vi "SelectColumnstoPlaybackDisplay_171213.vi"(11 "Clean data array in":dbl[][](array[numeric])) -> (0 "Speed":dbl[](array[numeric]), 1 "TotalDIstanceTraveled":dbl, 2 "Playbackprogress(min)maxscale":dbl, 3 "CurrentDIstancemaxScale":dbl, 4 "AVGSpeed":dbl, 5 "CurrentDistanceTraveled":dbl[](array[numeric]), 6 "TTL":dbl[](array[numeric]), 7 "Angle":dbl[](array[numeric]))   [LabVIEW 2016]
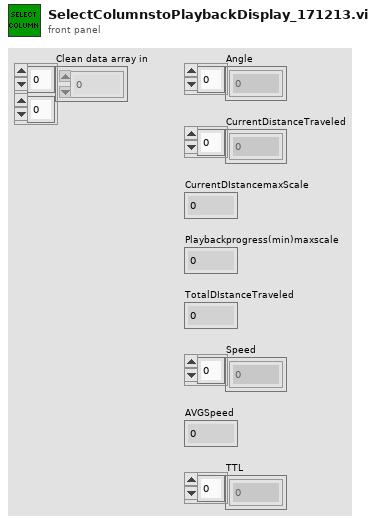
[diagram p1: front panel]
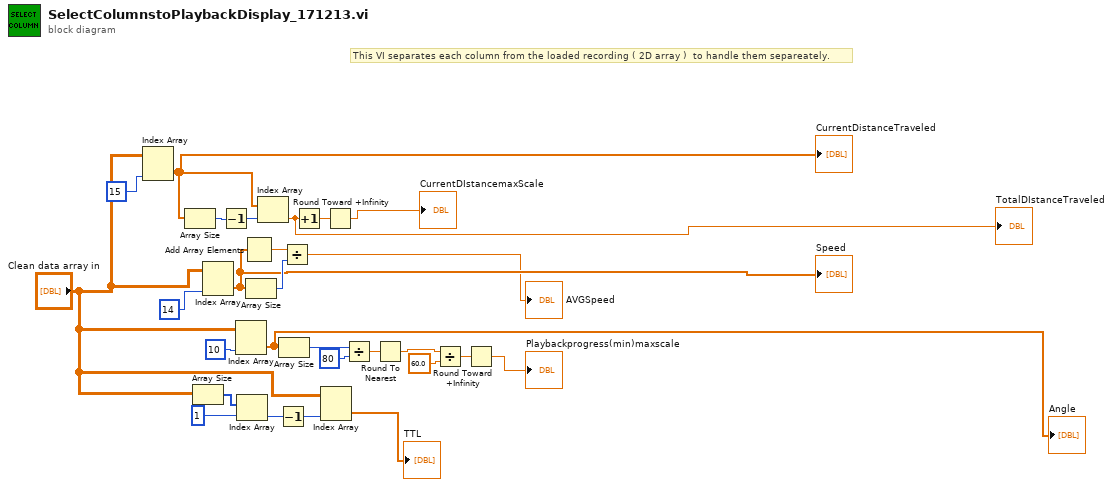
[diagram p0: block diagram]
diagram:
  # "This VI separates each column from the loaded recording ( 2D array )  to handle them separeately."
  n1 = Index Array(array="Clean data array in", index (col)=15 ("disabled index (col)")) -> (element=w5:dbl[])  [unwired: 1 in]
  "CurrentDistanceTraveled" <- w5
  n2 = Array Size(array=w5) -> (size(s)=w4:i32)
  n3 = Array Size(array="Clean data array in") -> (size(s)=w22:i32[])
  n4 = Index Array(array="Clean data array in", index (col)=14 ("disabled index (col)")) -> (element=w2:dbl[])  [unwired: 1 in]
  "Speed" <- w2
  n5 = Decrement(x=w4) -> (x-1=w3:i32)
  n6 = Index Array(array="Clean data array in", index (col)=10 ("disabled index (col)")) -> (element=w7:dbl[])  [unwired: 1 in]
  "Angle" <- w7
  n7 = Index Array(array=w22, index=1) -> (element=w25:i32)
  n8 = Add Array Elements(numeric array=w2) -> (sum=w12:dbl)
  n9 = Array Size(array=w2) -> (size(s)=w27:i32)
  n10 = Index Array(array=w5, index=w3) -> (element=w18:dbl)
  "TotalDIstanceTraveled" <- w18
  n11 = Decrement(x=w25) -> (x-1=w24:i32)
  n12 = Array Size(array=w7) -> (size(s)=w11:i32)
  n13 = Divide(x=w12, y=w27) -> (x/y=→"AVGSpeed":dbl)
  n14 = Increment(x=w18) -> (x+1=w20:dbl)
  n15 = Index Array(array="Clean data array in", index (col)=w24) -> (element=→"TTL":dbl[])  [unwired: 1 in]
  n16 = Round Toward +Infinity(x=w20) -> (ceil(x): smallest int >= x=→"CurrentDIstancemaxScale":dbl)
  n17 = Divide(x=w11, y=80) -> (x/y=w8:dbl)
  n18 = Round To Nearest(number=w8) -> (nearest integer value=w10:dbl)
  n19 = Divide(x=w10, y=60.0) -> (x/y=w9:dbl)
  n20 = Round Toward +Infinity(x=w9) -> (ceil(x): smallest int >= x=→"Playbackprogress(min)maxscale":dbl)
